vi "Perform Action.vi"(8 "error in (no error)":errorcluster, 10 "Input":variant, 11 "Virt Instrument Base in":refnum<class "Virt Voltage Generator.lvclass">) -> (0 "error out":errorcluster, 2 "Output":variant, 3 "Virt Instrument Base out":refnum<class "Virt Voltage Generator.lvclass">)   [LabVIEW 2023, in "Virt Instrs FGen.lvlib" / "Virt Voltage Generator.lvclass"]
uses:
  Virt Voltage Generator.lvclass
  D:/git/HAL/HAL GOOP4/Virtual Instrument Base/Virt Instr Base.lvclass
  FGen PXI/FGen PXI Std Waveform CFG/Std Waveform Action Pams.ctl
  Virtual Instrument Base/Virt Instr Base.lvclass/Virt Instr Base.ctl
  Virt Voltage Generator.lvclass/Virt Voltage Generator.ctl
  Virtual Instrument Base/Virt Instr Base.lvclass
  Instrument/Instrument.lvclass
  FGen PXI/FGen PXI Std Waveform CFG.lvlib
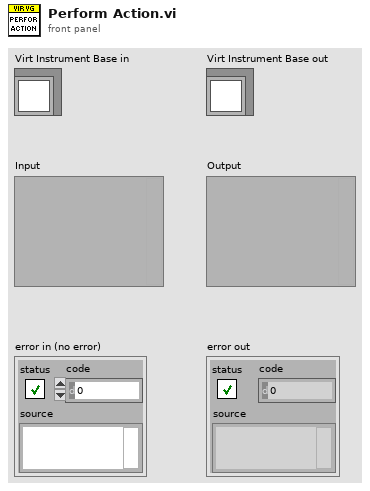
[diagram p1: front panel]
types:
  T1 = typedef "FGen PXI Std Waveform CFG.lvlib/Std Waveform Action Pams.ctl" = cluster{"Channel":string, "Std Waveform Pams":cluster{"Frequency":dbl, "Amplitude":dbl, "DC Offset":dbl}}
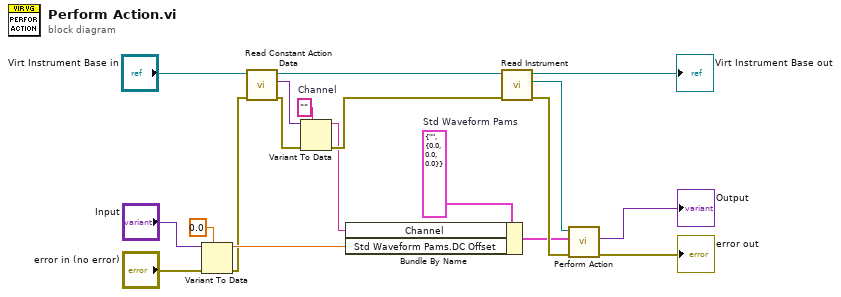
[diagram p0: block diagram]
diagram:
  w10 = ""  # Channel
  w19 = T1 {"Channel"="", "Std Waveform Pams"={"Frequency"=0.0, "Amplitude"=0.0, "DC Offset"=0.0}}  # Std Waveform Pams
  n1 = Variant To Data(error in="error in (no error)", type=0.0, Variant="Input") -> (data=w15:dbl, error out=w12:errorcluster)
  n2 = call "Read Constant Action Data.vi"("error in (no error)"=w12, "Virt Instrument Base in"="Virt Instrument Base in") -> ("error out"=w14:errorcluster, "Constant Action Data"=w9:variant, "Virt Instrument Base out"=w8:refnum<class "Virt Voltage Generator.lvclass">)  [unwired: 7 in]
  n3 = Variant To Data(error in=w14, type=w10, Variant=w9) -> (data=w2:string, error out=w11:errorcluster)
  n4 = Bundle By Name(cluster=w19, "Channel"=w2, "Std Waveform Pams.DC Offset"=w15) -> (w1:T1)
  n5 = call "Read Instrument.vi"("error in (no error)"=w11, "Virt Instr Base in"=w8) -> ("error out"=w6:errorcluster, "HAL GOOP4.lvlib:Instrument"=w7:refnum<class "Instrument.lvclass">, "Virt Instr Base out"=→"Virt Instrument Base out":refnum<class "Virt Voltage Generator.lvclass">)  [unwired: 7 in]
  n6 = call "Perform Action.vi"("Error In"=w6, "Input"=w1, "reference in"=w7) -> ("Error Out"=→"error out":errorcluster, "Output"=→"Output":variant)  [unwired: 6 in, 1 out]
